vi "Reset_Instr.vi"(8 "error in (no error)":errorcluster caption="entrée d'erreur (pas d'erreur)", 11 "Class Instrument Multimeter en entrée":refnum<class "Class Instrument LED_Analyser.lvclass">) -> (0 "error out":errorcluster caption="sortie d'erreur", 3 "Class Instrument Multimeter en sortie":refnum<class "Class Instrument LED_Analyser.lvclass">)   [LabVIEW 2020, in "Library Instrument & Equipement.lvlib" / "Library Instruments.lvlib" / "Class Instrument LED_Analyser.lvclass"]
uses:
  Class Instrument LED_Analyser.lvclass
  Class Instrument LED_Analyser.lvclass/Class Instrument LED_Analyser.ctl
  Instrument (Default)/Class Instrument (Default).lvclass
  LED Analyser/Class Led Analyser (Default)/Class LED Analyser (Default).lvclass
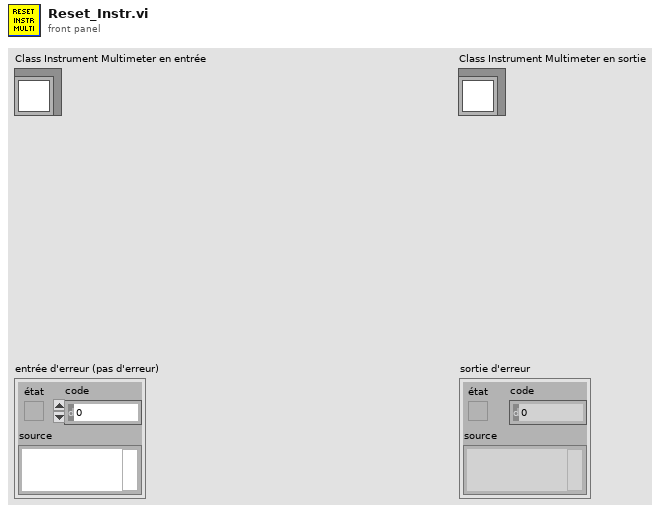
[diagram p1: front panel]
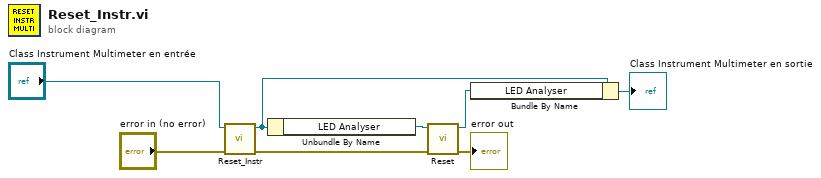
[diagram p0: block diagram]
diagram:
  n1 = call-parent "Reset_Instr.vi"("error in (no error)"="error in (no error)", "Class Instrument (Default) en entrée"="Class Instrument Multimeter en entrée") -> ("error out"=w4:errorcluster, "Class Instrument (Default) en sortie"=w6:refnum<class "Class Instrument LED_Analyser.lvclass">)  [unwired: 8 in]
  n2 = Unbundle By Name(w6) -> ("LED Analyser"=w2:refnum<class "Class LED Analyser (Default).lvclass">)
  n3 = call-dynamic "Reset.vi"("error in (no error)"=w4, "Class LED Analyser in"=w2) -> ("error out"=→"error out":errorcluster, "Class LED Analyser Out"=w1:refnum<class "Class LED Analyser (Default).lvclass">)  [unwired: 8 in]
  n4 = Bundle By Name(cluster=w6, "LED Analyser"=w1) -> (→"Class Instrument Multimeter en sortie":refnum<class "Class Instrument LED_Analyser.lvclass">)
